vi "Get Motion Done (SubVI).vi"(0 "CmdLib In":refnum<k24>, 1 "DeviceKey In":string, 2 "Device Address In":i32, 3 "Motor":i32, 4 "done":bool, 5 "error in (no error)":errorcluster) -> (14 "CmdLib Out":refnum<k24>, 15 "DeviceKey Out":string, 17 "Device Address Out":i32, 18 "Is Motion Done":bool, 19 "error out":errorcluster)   [LabVIEW 2017]
doc: "by Tanguy BOULARD"
uses:
  dll/CmdLib.dll
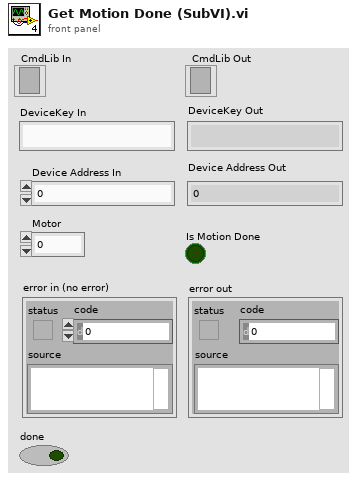
[diagram p1: front panel]
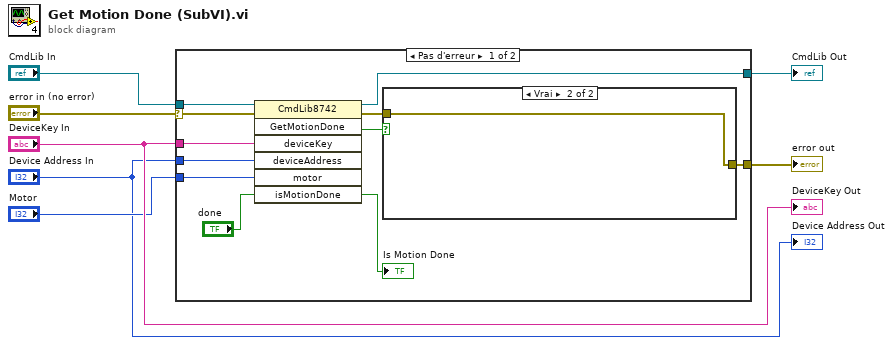
[diagram p0: block diagram]
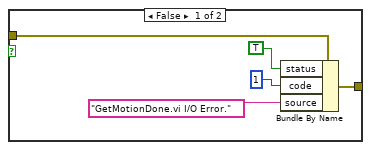
[diagram p2: hidden frame]
diagram:
  n1 = case shown="Pas d'erreur" "error in (no error)" {
    selector: "error in (no error)" -> [w8 w26]
    tunnel: "CmdLib In" -> [w18 w25]
    tunnel: [w17 w25] -> w6
    tunnel: "DeviceKey In" -> [w16 _]
    tunnel: [w15 w26] -> w4
    tunnel: "Motor" -> [w14 _]
    tunnel: "Device Address In" -> [w13 _]
    frame No Error {
      n2 = invoke class="CmdLib8742" method="GetMotionDone"(reference=w18, error in=w8, "deviceKey"=w16, "deviceAddress"=w13, "motor"=w14, "isMotionDone"="done") -> (reference out=w17:refnum<k24>, error out=w11:errorcluster, "GetMotionDone"=w12:bool, "isMotionDone"=→"Is Motion Done":bool)  [unwired: 1 in, 3 out]
      n3 = case shown="Vrai" w12 {
        tunnel: w11 -> [w23 w24]
        tunnel: [w22 w24] -> w15
        frame False {
          n4 = Bundle By Name(cluster=w23, "status"=TRUE, "code"=1, "source"="GetMotionDone.vi I/O Error.") -> (w22:errorcluster)
        }
        frame True {
        }
      }
    }
    frame Error {
    }
  }
  "error out" <- w4
  "CmdLib Out" <- w6
  "DeviceKey Out" <- "DeviceKey In"
  "Device Address Out" <- "Device Address In"
